vi "Save JSON File.vi"(8 "error in (no error)":errorcluster, 10 "Data":variant, 11 "Control Experiment in":refnum<class "Control Experiment.lvclass">) -> (0 "error out":errorcluster)   [LabVIEW 2019, in "Control Experiment.lvclass"]
uses:
  Control Experiment.lvclass
  Control Experiment.lvclass/Control Experiment.ctl
  <vilib>/addons/_JKI.lib/Serialization/JSON/JKI JSON Serialization.lvlib
panel:
  out "Control Experiment out":refnum<class "Control Experiment.lvclass">
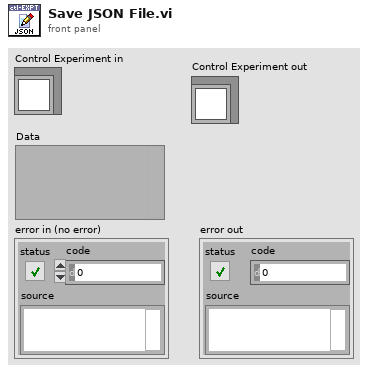
[diagram p1: front panel]
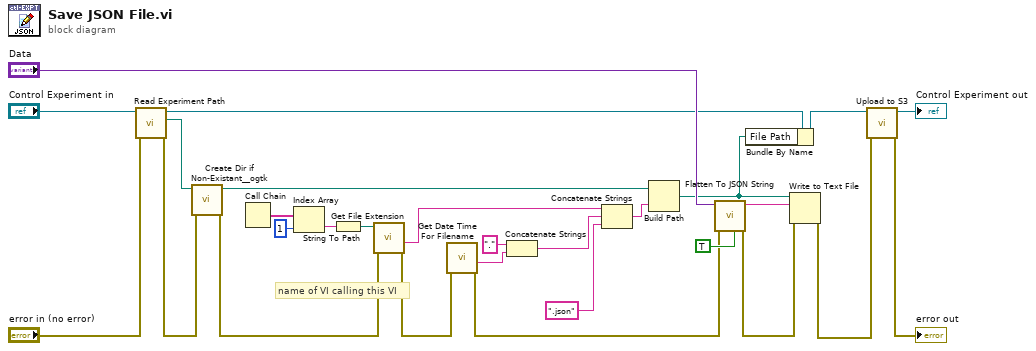
[diagram p0: block diagram]
diagram:
  # "name of VI calling this VI"
  n1 = call "Read Experiment Path.vi"("error in (no error)"="error in (no error)", "Control Experiment in"="Control Experiment in") -> ("error out"=w19:errorcluster, "Experiment Path"=w16:path, "Control Experiment out"=w8:refnum<class "Control Experiment.lvclass">)  [unwired: 7 in]
  n2 = call <userlib>:"Create Dir if Non-Existant__ogtk.vi"("error in (no error)"=w19, "Directory Path"=w16) -> ("error out"=w14:errorcluster, "dup Directory Path"=w9:path)  [unwired: 7 in, 1 out]
  n3 = Call Chain() -> (call chain=w25:string[])
  n4 = Index Array(array=w25, index=1) -> (element=w26:string)
  n5 = String To Path(string=w26) -> (path=w28:path)
  n6 = call <vilib>:"Get File Extension.vi"("error in (no error)"=w14, "file"=w28) -> ("error out"=w1:errorcluster, "filename without extension"=w13:string)  [unwired: 5 in, 3 out]
  n7 = call "Get Date Time For Filename.vi"("error in (no error)"=w1) -> ("error out"=w2:errorcluster, "date-time string"=w11:string)  [unwired: 8 in, 1 out]
  n8 = Concatenate Strings("." ("string"), w11) -> (w10:string)
  n9 = Concatenate Strings(w13, w10, ".json" ("string")) -> (w23:string)
  n10 = Build Path(base path=w9, name or relative path=w23) -> (appended path=w7:path)
  n11 = call <vilib>:"Flatten To JSON String.vi"("Enums As String (F)"=TRUE, "error in (no error)"=w2, "Variant"="Data") -> ("error out"=w18:errorcluster, "JSON String"=w22:string)  [unwired: 7 in]
  n12 = Bundle By Name(cluster=w8, "File Path"=w7) -> (w6:refnum<class "Control Experiment.lvclass">)
  n13 = Write to Text File(file (use dialog)=w7, text=w22, error in=w18) -> (error out=w5:errorcluster)  [unwired: 1 in, 2 out]
  n14 = call "Upload to S3.vi"("error in (no error)"=w5, "Control Experiment in"=w6) -> ("error out"=→"error out":errorcluster, "Control Experiment out"=→"Control Experiment out":refnum<class "Control Experiment.lvclass">)  [unwired: 8 in]
